vi "Task_Enum.vi"(8 "error in (no error)":errorcluster caption="错误输入（无错误）", 10 "Enum":T1(ring), 11 "zsActor输入":refnum<class "ActorWrapper.lvclass">) -> (0 "error out":errorcluster caption="错误输出", 3 "zsActor输出":refnum<class "ActorWrapper.lvclass">)   [LabVIEW 2014, in "Wrapper.lvlib" / "ActorWrapper.lvclass"]
uses:
  ActorWrapper.lvclass
  ActorWrapper.lvclass/ActorWrapper.ctl
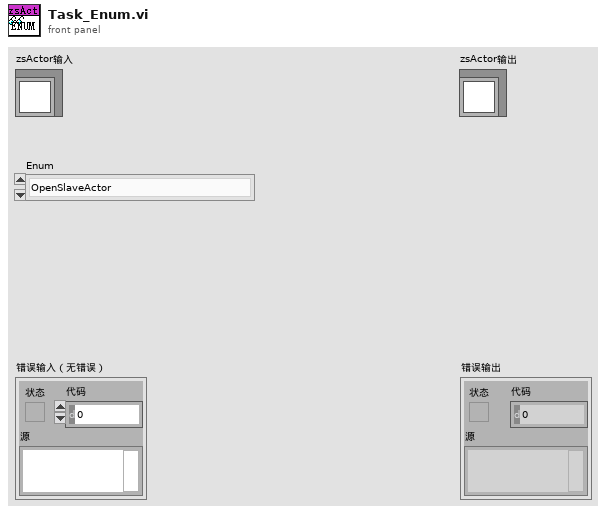
[diagram p1: front panel]
types:
  T1 = enum16{"OpenSlaveActor", "Idle", "StopSlaveActor"}
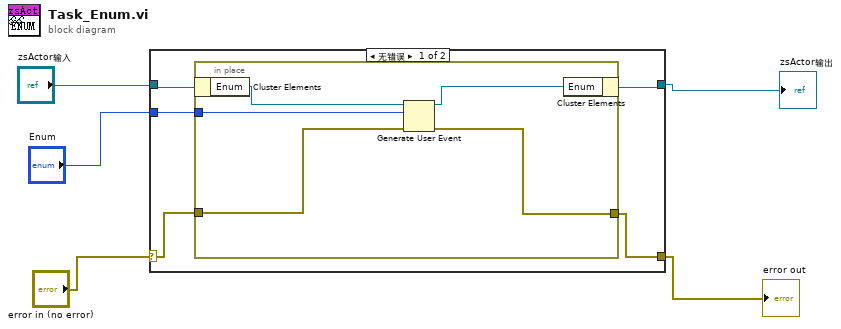
[diagram p0: block diagram]
diagram:
  n1 = case shown="无错误" "error in (no error)" {
    selector: "error in (no error)" -> [w8 w16]
    tunnel: [w7 w16] -> w2
    tunnel: [w6 w17] -> w5
    tunnel: "zsActor输入" -> [w10 w17]
    tunnel: "Enum" -> [w9 _]
    frame No Error {
      n2 = in-place {
        in-place-border: w8 -> [w13]
        in-place-border: [w12] -> w7
        in-place-border: w9 -> [w11]
        n3 = in-place-cluster #1(w10) -> ("Enum"=w15:refnum<user-event>)
        n4 = Generate User Event(user event=w15, event data cluster=w11, error in=w13) -> (user event out=w14:refnum<user-event>, error out=w12:errorcluster)  [unwired: 1 in]
        n5 = in-place-cluster #1("Enum"=w14) -> (w6:refnum<class "ActorWrapper.lvclass">)
      }
    }
    frame Error {
    }
  }
  "error out" <- w2
  "zsActor输出" <- w5
